vi "Create Launch Notifier.vi"(8 "error in (no error)":errorcluster, 11 "Actor in":refnum<class "Actor.lvclass">) -> (0 "error out":errorcluster, 3 "Actor out":refnum<class "Actor.lvclass">)   [LabVIEW 2015, in "Actor.lvclass"]
uses:
  Actor.lvclass
  Actor.lvclass/Actor.ctl
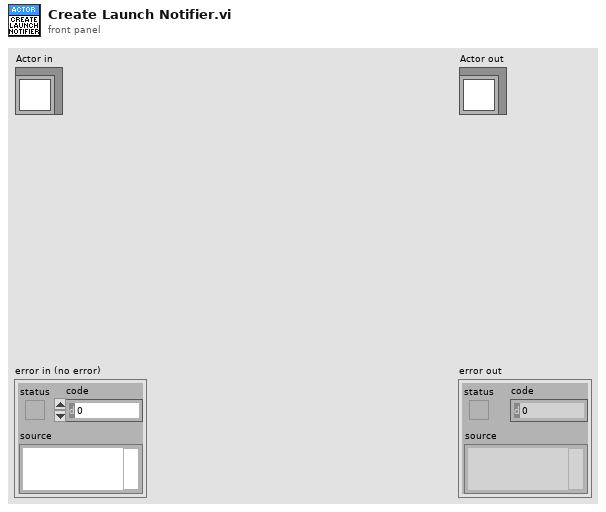
[diagram p1: front panel]
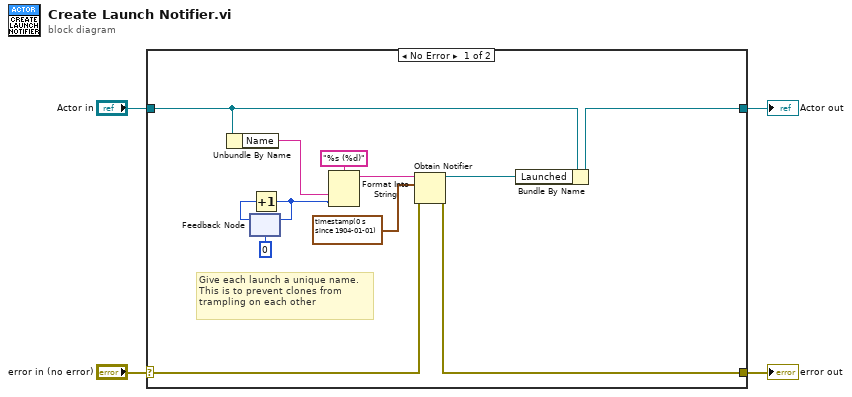
[diagram p0: block diagram]
diagram:
  n1 = case shown="No Error" "error in (no error)" {
    selector: "error in (no error)" -> [w16 w18]
    tunnel: [w15 w18] -> w3
    tunnel: [w6 w17] -> w1
    tunnel: "Actor in" -> [w7 w17]
    frame No Error {
      # "Give each launch a unique name. This is to prevent clones from trampling on each other"
      n2 = Unbundle By Name(w7) -> ("Name"=w11:string)
      n3 = feedback #1(0) -> (w13:i32)
      n4 = Increment(x=w13) -> (x+1=w10:i32)
      n5 = feedback-in #1(w10) -> ()
      n6 = Format Into String(format string="%s (%d)", w11, w10) -> (resulting string=w9:string)  [unwired: 2 in, 1 out]
      n7 = Obtain Notifier(name (unnamed)=w9, notification data type=timestamp(0 s since 1904-01-01), error in (no error)=w16) -> (notifier out=w5:refnum<notifier>, error out=w15:errorcluster)  [unwired: 1 in, 1 out]
      n8 = Bundle By Name(cluster=w7, "Launched"=w5) -> (w6:refnum<class "Actor.lvclass">)
    }
    frame Error {
    }
  }
  "error out" <- w3
  "Actor out" <- w1
